vi "Motic Open Camera.vi"(8 "error in (no error)":errorcluster, 11 "camera":i32) -> (0 "error out":errorcluster, 3 "camera out":i32)   [LabVIEW 2012, in "MoticApi.lvlib"]
doc: "MOTICAPI bool Motic_OpenCamera(MUCam_Handle camera);"
uses:
  MoticApi.lvlib
  MoticApi.dll
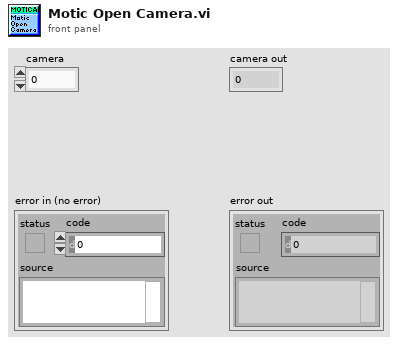
[diagram p1: front panel]
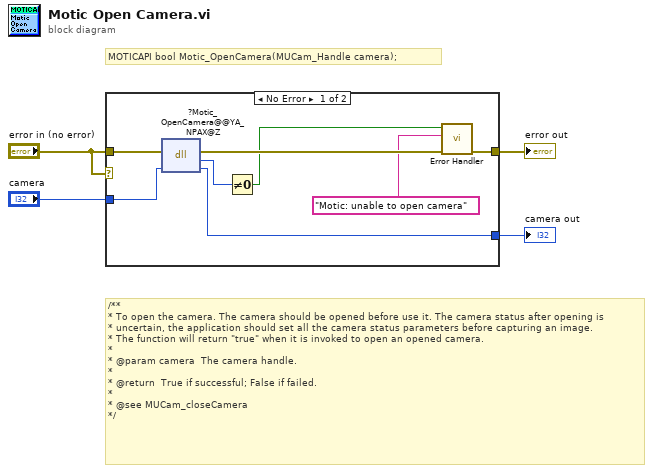
[diagram p0: block diagram]
diagram:
  # "/**\n* To open the camera. The camera should be opened before use it. The camera status after opening is\n* uncertain, the application should set all the camera status parameters before capturing an image.\n* The function will return \"true\" when it is invoked to open an opened camera.\n*\n* @param camera  The camera handle.\n*\n* @return  True if successful; False if failed.\n*\n* @see MUCam_closeCamera\n*/"
  # "MOTICAPI bool Motic_OpenCamera(MUCam_Handle camera);"
  n1 = case shown="No Error" "error in (no error)" {
    tunnel: "camera" -> [w11 w13]
    tunnel: [w10 w13] -> w3
    tunnel: "error in (no error)" -> [w9 w14]
    tunnel: [w7 w14] -> w2
    frame No Error {
      n2 = dll-call lib="C:/Users/TTS-Digital/Desktop/MoticApi/MoticApi_git/MoticApi/MoticApi.*" fn="?Motic_OpenCamera@@YA_NPAX@Z"(error in=w9, "camera"=w11) -> (error out=w8:errorcluster, "return type"=w12:u8, "camera"=w10:i32)  [unwired: 2 in, 1 out]
      n3 = Not Equal To 0?(x=w12) -> (x != 0?=w6:bool)
      n4 = call "Error Handler.vi"("error in (no error)"=w8, "Error message"="Motic: unable to open camera" ("source"), "Function return"=w6) -> ("error out"=w7:errorcluster)  [unwired: 8 in]
    }
    frame Error {
    }
  }
  "camera out" <- w3
  "error out" <- w2
